vi "NCD Update Settings Valve.vi"(8 "error in (no error)":errorcluster, 10 "Message Data":variant, 11 "Data Cluster":T1={"MFC Definition"={"MFC Port"="", "MFC Enable"=TRUE, "Baud Rate"=0, "Interface type"=enum."RS-485", "Address"=0}, "Set Point Options"={"Setpoint Value"=0.0, "Mass Flow EU 2"="", "Setpoint Source"="", "Valve Mode"=""}, "Writer Queue"=refnum, "Enable"=FALSE, "Update Rate"=0, "MRC Chamber Enable"=FALSE, "Selected Gas"="", "Address String"=""} {"Set Point Options"."Setpoint Value" min=0.0 max=0.62495 format="%.5f"}) -> (0 "error out":errorcluster, 2 "Send Resp":bool, 3 "Data Cluster out":T1={"MFC Definition"={"MFC Port"="", "MFC Enable"=TRUE, "Baud Rate"=0, "Interface type"=enum."RS-485", "Address"=0}, "Set Point Options"={"Setpoint Value"=0.0, "Mass Flow EU 2"="", "Setpoint Source"="", "Valve Mode"=""}, "Writer Queue"=refnum, "Enable"=FALSE, "Update Rate"=0, "MRC Chamber Enable"=FALSE, "Selected Gas"="", "Address String"=""} {"Set Point Options"."Setpoint Value" min=0.0 max=0.62495 format="%.5f"})   [LabVIEW 2020]
uses:
  MRC Configuration.ctl
  support/Message Queue/Message Cluster.ctl
  support/HW Message Cluster.ctl
  support/Message Queue/Message Queue.lvlib
  MRC Module.lvlib
panel:
  out "Status":string
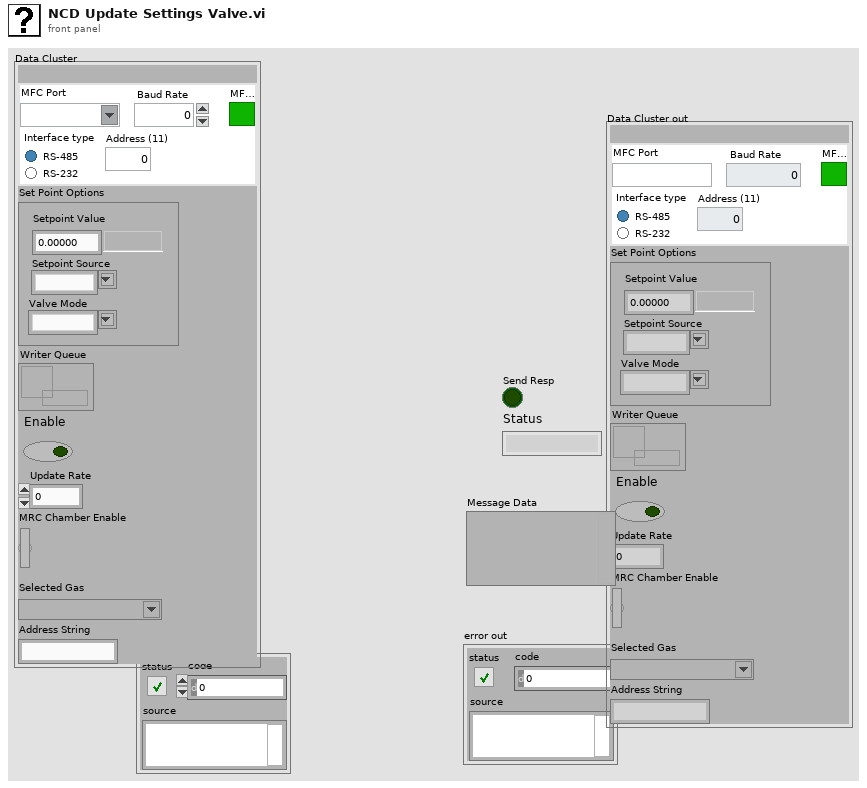
[diagram p1: front panel]
types:
  T1 = typedef "MRC Module.lvlib/MRC Configuration.ctl" = cluster{"MFC Definition":cluster{"MFC Port":refnum<visa-resource-name>, "MFC Enable":bool, "Baud Rate":i32, "Interface type":enum32{"RS-485", "RS-232"}, "Address":i32}, "Set Point Options":cluster{"Setpoint Value":dbl, "Mass Flow EU 2":string, "Setpoint Source":string, "Valve Mode":string}, "Writer Queue":refnum<queue>, "Enable":bool, "Update Rate":u32, "MRC Chamber Enable":bool, "Selected Gas":string, "Address String":string}
  T2 = typedef "Message Queue.lvlib/HW Message Cluster.ctl" = cluster{"Writer Queue":refnum<queue>, "Writer Data":T3}
  T3 = typedef "Message Queue.lvlib/Message Cluster.ctl" = cluster{"Message":string, "Message Data":variant}
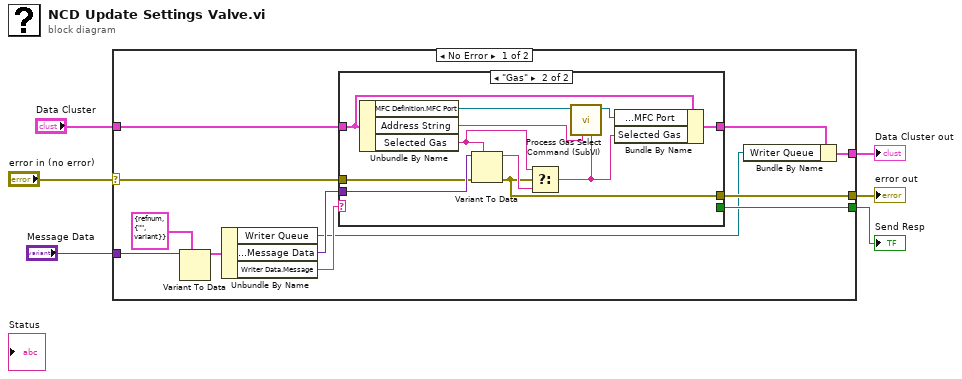
[diagram p0: block diagram]
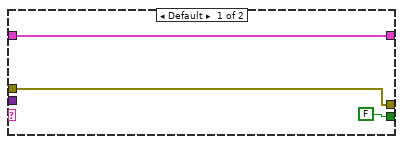
[diagram p2: hidden frame]
diagram:
  n1 = case shown="No Error" "error in (no error)" {
    selector: "error in (no error)" -> [w12 w33]
    tunnel: [w18 w33] -> w6
    tunnel: "Data Cluster" -> [w17 w34]
    tunnel: [w9 w34] -> w4
    tunnel: "Message Data" -> [w13 _]
    tunnel: [w10 _] -> w1
    frame No Error {
      n2 = Variant To Data(type=T2 {"Writer Queue"=refnum, "Writer Data"={"Message"="", "Message Data"=variant}}, Variant=w13) -> (data=w14:T2)  [unwired: 1 in, 1 out]
      n3 = Unbundle By Name(w14) -> ("Writer Queue"=w8:refnum<queue>, "Writer Data.Message Data"=w11:variant, "Writer Data.Message"=w15:string)
      n4 = case shown="\"Gas\"" w15 {
        tunnel: w11 -> [_ w31]
        tunnel: [w21 w30] -> w16
        tunnel: w17 -> [w21 w32]
        tunnel: w12 -> [w20 w27]
        tunnel: [w20 w26] -> w18
        tunnel: [FALSE ("Send Resp") _] -> w10
        frame Default {
        }
        frame "Gas" {
          n5 = Unbundle By Name(w32) -> ("MFC Definition.MFC Port"=w24:refnum<visa-resource-name>, "Address String"=w25:string, "Selected Gas"=w29:string)
          n6 = Variant To Data(error in=w27, type=w29, Variant=w31) -> (data=w28:string, error out=w26:errorcluster)
          n7 = Select(t=w29, s=w26, f=w28) -> (s? t:f=w22:string)
          n8 = call "Process Gas Select Command (SubVI).vi"("Gas Select In"=w22, "Address"=w25, "VISA Refnum in"=w24) -> ("VISA Refnum out"=w23:refnum<visa-resource-name>)  [unwired: 6 in, 2 out]
          n9 = Bundle By Name(cluster=w32, "MFC Definition.MFC Port"=w23, "Selected Gas"=w22) -> (w30:T1)
        }
      }
      n10 = Bundle By Name(cluster=w16, "Writer Queue"=w8) -> (w9:T1)
    }
    frame Error {
    }
  }
  "error out" <- w6
  "Data Cluster out" <- w4
  "Send Resp" <- w1
